vi "Serial_Global.vi"() -> ()   [LabVIEW 2020]
panel:
  in  "pause?":bool
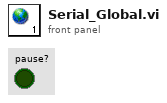
[diagram p1: front panel]
diagram:
